vi "keccak.ip.test.wrapper.vi"() -> ()   [LabVIEW 2021]
uses:
  <vilib>/Platform/TimedLoop/XDataNode/timing_clust.ctl
  <vilib>/Platform/TimedLoop/XDataNode/nitl_modes.ctl
  <vilib>/Platform/TimedLoop/XDataNode/wakeup.ctl
  <vilib>/rvi/Emulation/niFpgaSctlEmulationGetInTimedLoop.vi
  <vilib>/rvi/Emulation/niFpgaEmulationReportErrorSimple.vi
  <vilib>/rvi/Emulation/niFpgaGetClockAttributes.vi
  <vilib>/rvi/Emulation/niFpgaCriticalErrorInLSC.vi
  <vilib>/rvi/interface/RandomDataEmulation/niFpgaRandomDataHandleErrors.vi
  <vilib>/rvi/DataTransferAndStorage/Container/Common/niFpgaContainerExecOnDevCompGetState.vi
  <vilib>/rvi/Emulation/niFpgaEmulationIsFPGAContextNoSignature.vi
  <vilib>/rvi/errors/niFpgaSetErrorForExecOnDevCompSimple.vi
  <vilib>/rvi/eio/common/nirviEmuReportErrorAndStop.vi
  <vilib>/rvi/DataTransferAndStorage/Container/Common/niFpgaContainerGetUniqueNameForEmu.vi
  <vilib>/rvi/FIFO/Fifo_Resource/nirvififoEmulationSetSize.vi
  <vilib>/rvi/FIFO/Fifo_Resource/nirviFifoEmulationQueueMgr.vi
  <instcachedir>/0/nirviFifoEmulationQueueMgr_E5CAEC123FF24DC58D834DCA3CDAA9B5.lvgen/nirviFifoEmulationQueueMgr_E5CAEC123FF24DC58D834DCA3CDAA9B5_000.vi
  <vilib>/rvi/FIFO/Fifo_Resource/nirvififoEmulationDetermineInputValidOut.vi
  <vilib>/rvi/FIFO/Fifo_Resource/nirvififoEmulationCreateLock.vi
  <vilib>/rvi/Emulation/niFpgaProcessEmulError.vi
  <vilib>/rvi/FIFO/Fifo_Resource/nirvififoEmulationObtainLock.vi
  <vilib>/rvi/FIFO/Fifo_Resource/nirvififoEmulationReleaseLock.vi
  <vilib>/rvi/occurrence/nirviWaitOnOccurrenceBase.vi
  <vilib>/rvi/errors/nirviReportUnexpectedCaseInternalError.vi
  <vilib>/rvi/errors/nirviReportUnexpectedCaseInternalError (U32).vi
  <vilib>/Utility/error.llb/Clear Errors.vi
  <vilib>/platform/TimedLoop/XDataNode/XDataNode.xnode
  <vilib>/rvi/DataTransferAndStorage/Container/XNode/niFpgaContainer.xnode
  <vilib>/rvi/interface/RandomDataEmulation/nirviRandomDataFpgaReadWriteTemplate.vi
  <vilib>/rvi/FIFO/Fifo_Resource/niFpgaFifoEmulationRefIn.vi
  <vilib>/Platform/TimedLoop/XDataNode/XDNodeRunTimeDep.lvlib
panel:
  in  "Reset":bool
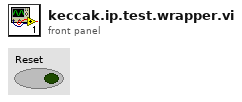
[diagram p1: front panel]
types:
  T1 = cluster{"TS_PARMS":refnum<k21>, "TS_DATA":refnum<k21>, "TS_RESULTS":refnum<k21>}
  T2 = typedef "XDNodeRunTimeDep.lvlib/timing_clust.ctl" = cluster{"Expected End [f-1]":u64, "Actual End [f-1]":u64, "Finished Late? [f-1]":bool, "Expected End [i-1]":u64, "Actual End [i-1]":u64, "Finished Late? [i-1]":bool, "Expected Start [i]":u64, "Actual Start [i]":u64, "Expected Start [f]":u64, "Actual Start [f]":u64, "Source Name":string, "Structure Name":string, "Period":i64, "Deadline":i64, "Offset":i64, "Start":i64, "Priority":i32, "Timeout":i32, "Mode":T3, "Wakeup Reason":T4, "Error":errorcluster, "Source Type":string, "Secondary Source Type":string, "Global End Time":u64, "Global Start Time":u64, "Frame Duration":u64, "Iteration Duration":u64, "Assigned CPU":i32, "I/O Scan Engine Mode":u32}
  T3 = typedef "XDNodeRunTimeDep.lvlib/nitl_modes.ctl" = enum32{"No Change", "Process missed periods, maintain original phase", "Discard missed periods, maintain original phase", "Process missed periods, ignore original phase", "Discard missed periods, ignore original phase"}
  T4 = typedef "XDNodeRunTimeDep.lvlib/wakeup.ctl" = enum32{"Normal", "Aborted", "Asynchronous wakeup", "Timing source error", "Timed loop error", "Timeout"}
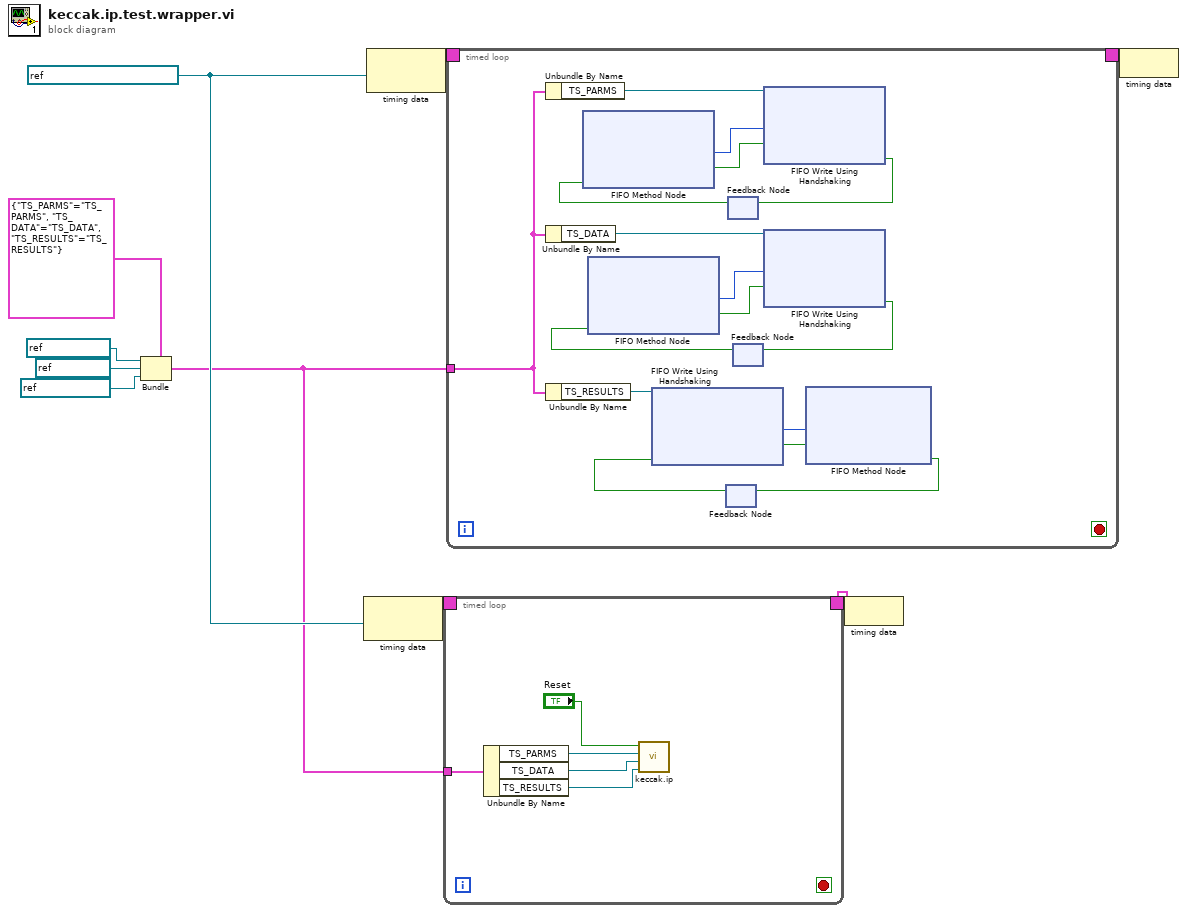
[diagram p0: block diagram]
diagram:
  w6 = refnum<k21> "40 MHz Onboard Clock" ("Source Name")
  n1 = Bundle(cluster=T1 {"TS_PARMS"="TS_PARMS", "TS_DATA"="TS_DATA", "TS_RESULTS"="TS_RESULTS"}, "TS_PARMS"=refnum<k21> "TS_PARMS" ("FIFO.RESULTS"), "TS_DATA"=refnum<k21> "TS_DATA" ("FIFO.RESULTS"), "TS_RESULTS"=refnum<k21> "TS_RESULTS" ("FIFO.RESULTS")) -> (w5:T1)
  n2 = node-c288(w6) -> (w8:T2)
  n3 = node-c288(w6) -> (w10:T2)
  n4 = timed-loop {
    timing: w8 -> [_]
    timing-out: [_] -> w7
    tunnel: w5 -> [w14]
    stop <- _ stop-if-true
    n5 = Unbundle By Name(w14) -> ("TS_PARMS"=w13:refnum<k21>, "TS_DATA"=w12:refnum<k21>, "TS_RESULTS"=w11:refnum<k21>)
    n6 = call "keccak.ip.vi"("FIFO.RESULTS"=w11, "FIFO.DATA"=w12, "FIFO.PARMS"=w13, "Reset"="Reset") -> ()  [unwired: 8 in]
  }
  n7 = timed-loop {
    timing: w10 -> [_]
    timing-out: [_] -> w9
    tunnel: w5 -> [w31]
    stop <- _ stop-if-true
    n8 = Unbundle By Name(w31) -> ("TS_PARMS"=w33:refnum<k21>)
    n9 = Unbundle By Name(w31) -> ("TS_DATA"=w32:refnum<k21>)
    n10 = Unbundle By Name(w31) -> ("TS_RESULTS"=w30:refnum<k21>)
    n11 = feedback #1() -> (w18:bool)  [unwired: 1 in]
    n12 = xnode ("FIFO Write Using Handshaking")("Ready for Output"=w18, "FIFO In"=w30) -> ("Element"=w21:u64, "Output Valid"=w20:bool)  [unwired: 1 out]
    n13 = feedback #2() -> (w26:bool)  [unwired: 1 in]
    n14 = xnode ("FIFO Method Node")("Ready for Output"=w26) -> ("Element"=w29:u64, "Output Valid"=w28:bool)  [unwired: 1 in, 1 out]
    n15 = feedback #3() -> (w22:bool)  [unwired: 1 in]
    n16 = xnode ("FIFO Method Node")("Ready for Output"=w22) -> ("Element"=w25:u64, "Output Valid"=w24:bool)  [unwired: 1 in, 1 out]
    n17 = xnode ("FIFO Write Using Handshaking")("Element"=w29, "Input Valid"=w28, "FIFO In"=w33) -> ("Ready for Input"=w27:bool)  [unwired: 1 out]
    n18 = feedback-in #2(w27) -> ()
    n19 = xnode ("FIFO Write Using Handshaking")("Element"=w25, "Input Valid"=w24, "FIFO In"=w32) -> ("Ready for Input"=w23:bool)  [unwired: 1 out]
    n20 = feedback-in #3(w23) -> ()
    n21 = xnode ("FIFO Method Node")("Element"=w21, "Input Valid"=w20) -> ("Ready for Input"=w19:bool)  [unwired: 1 in, 1 out]
    n22 = feedback-in #1(w19) -> ()
  }
  n23 = node-c288(w7) -> ()
  n24 = node-c288(w9) -> ()
